vi "FTW-TestExecutive-Core_StepTypes_Define.vi"(0 "FTW-TestExecutive-Core In":refnum<class "FTW-TestExecutive-Core.lvclass">, 11 "error in":errorcluster) -> (4 "FTW-TestExecutive-Core Out":refnum<class "FTW-TestExecutive-Core.lvclass">, 15 "error out":errorcluster)   [LabVIEW 2015, in "FTW-TestExecutive-Core.lvclass"]
uses:
  FTW-TestExecutive-Core.lvclass
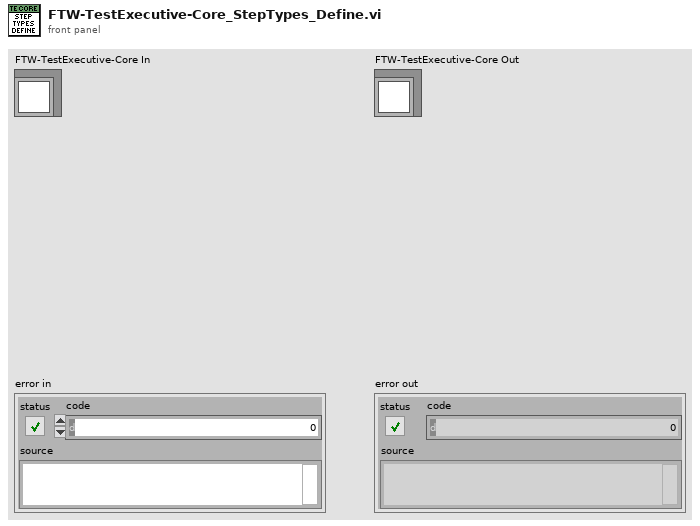
[diagram p1: front panel]
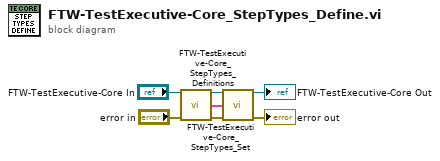
[diagram p0: block diagram]
diagram:
  n1 = call-dynamic "FTW-TestExecutive-Core_StepTypes_Definitions.vi"("FTW-TestExecutive-Core In"="FTW-TestExecutive-Core In", "error in"="error in") -> ("FTW-TestExecutive-Core Out"=w2:refnum<class "FTW-TestExecutive-Core.lvclass">, "Step Types"=w1:cluster{"Name":string, "Base Config":string}[], "error out"=w4:errorcluster)  [unwired: 11 in]
  n2 = call "FTW-TestExecutive-Core_StepTypes_Set.vi"("FTW-TestExecutive-Core In"=w2, "Step Types"=w1, "error in"=w4) -> ("FTW-TestExecutive-Core Out"=→"FTW-TestExecutive-Core Out":refnum<class "FTW-TestExecutive-Core.lvclass">, "error out"=→"error out":errorcluster)  [unwired: 11 in]
